vi "spindle_power_save.vi"(0 "Byte Stream File in":refnum<file>, 2 "Array":dbl[](array[numeric]), 5 "base path":path, 7 "Record  SS 661":bool, 9 "Boolean 3":bool, 11 "error in (no error)":errorcluster) -> (4 "Byte Stream File out":refnum<file>, 6 "Boolean 2":bool, 15 "error out":errorcluster)   [LabVIEW 2014]
panel:
  out "Array 2":dbl[](array[numeric])
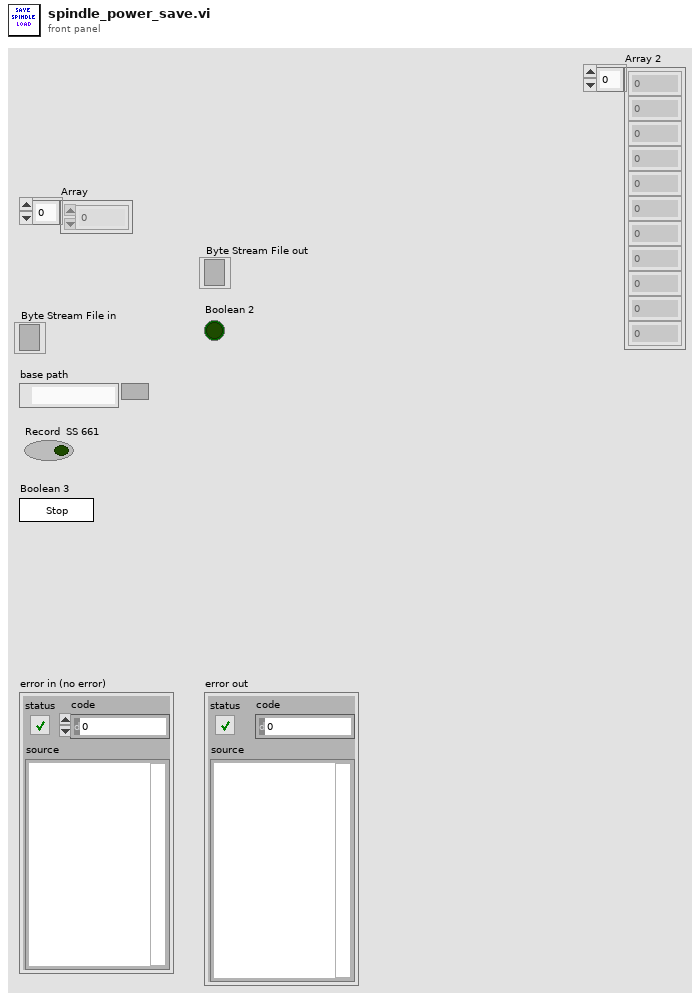
[diagram p1: front panel]
types:
  T1 = enum16{"NotSaving", "Create", "Reading", "Closing"}
  T2 = cluster{"Array":dbl[], "seconds since 1Jan1904":timestamp}
  T3 = enum16{"open", "replace", "create", "open or create", "replace or create", "replace or create with confirmation"}
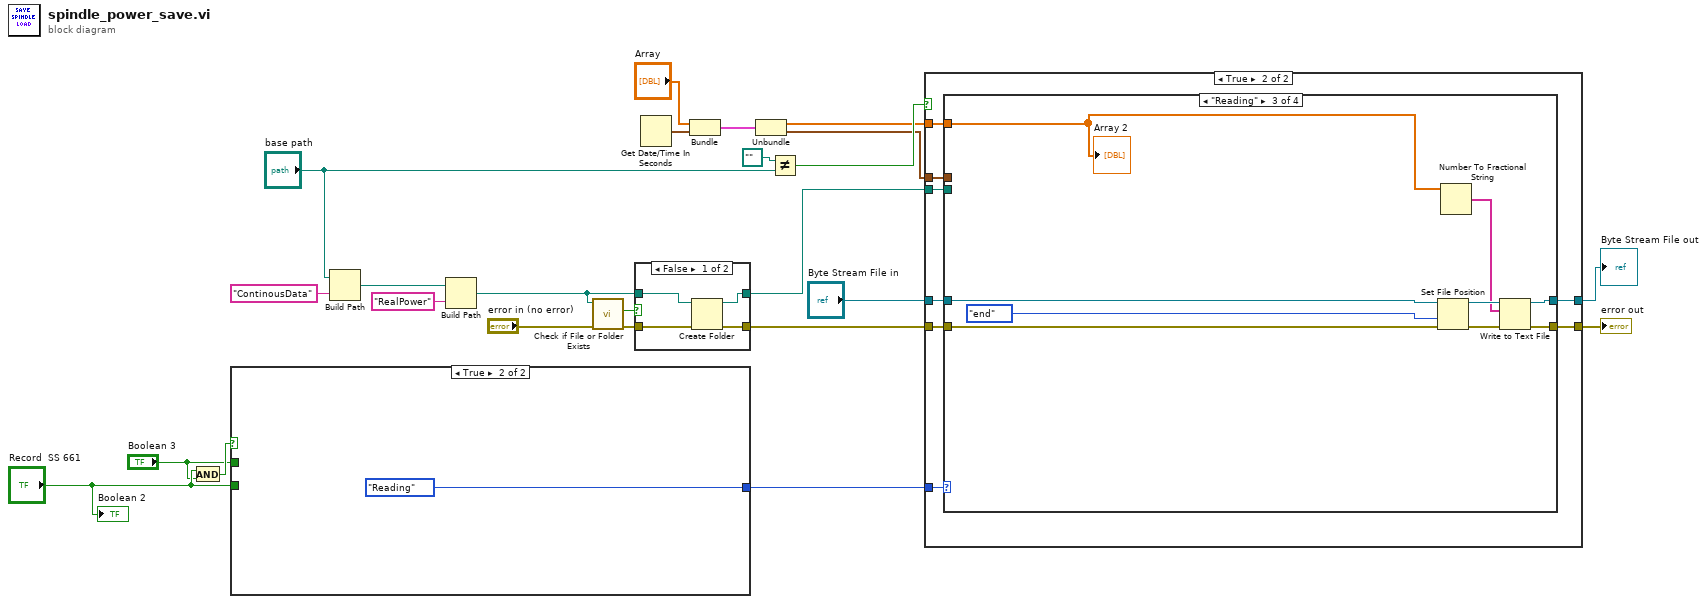
[diagram p0: block diagram]
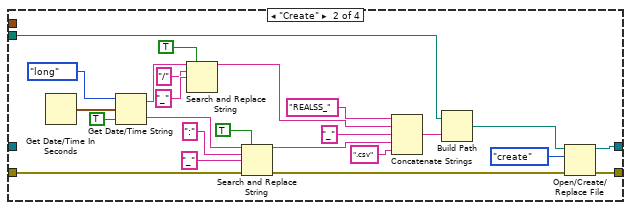
[diagram p5: hidden frame]
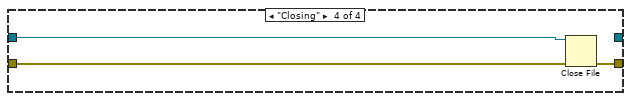
[diagram p6: hidden frame]
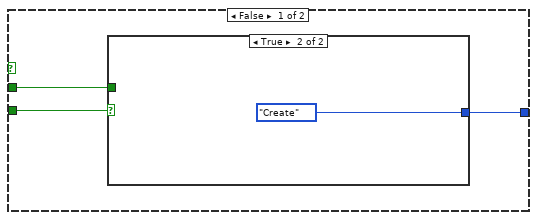
[diagram p7: hidden frame]
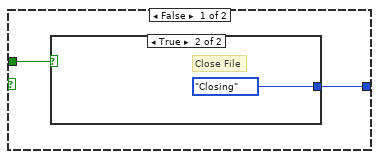
[diagram p8: hidden frame]
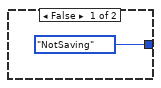
[diagram p9: hidden frame]
diagram:
  n1 = And(x="Record  SS 661", y="Boolean 3") -> (x .and. y?=w18:bool)
  n2 = case shown="True" w18 {
    tunnel: "Boolean 3" -> [w27 _]
    tunnel: [w26 T1."Reading" ("Enum")] -> w17
    tunnel: "Record  SS 661" -> [w25 _]
    frame False {
      n3 = case shown="True" w25 {
        tunnel: w27 -> [w29 _]
        tunnel: [w28 T1."Create" ("Enum")] -> w26
        frame False {
          n4 = case shown="True" w29 {
            tunnel: [T1."NotSaving" ("Enum") T1."Closing" ("Enum")] -> w28
            frame False {
            }
            frame True {
              # "Close File"
            }
          }
        }
        frame True {
        }
      }
    }
    frame True {
    }
  }
  n5 = Build Path(base path="base path", name or relative path="ContinousData") -> (appended path=w9:path)
  n6 = Build Path(base path=w9, name or relative path="RealPower") -> (appended path=w8:path)
  n7 = call <vilib>:"Check if File or Folder Exists.vi"("error in (no error)"="error in (no error)", "path"=w8) -> ("error out"=w11:errorcluster, "file or folder exists?"=w12:bool)  [unwired: 7 in, 1 out]
  n8 = case shown="False" w12 {
    tunnel: [w37 w39] -> w6
    tunnel: w11 -> [w36 w39]
    tunnel: w8 -> [w35 w38]
    tunnel: [w34 w38] -> w7
    frame False {
      n9 = Create Folder(path (use dialog)=w35, error in=w36) -> (created path=w34:path, error out=w37:errorcluster)  [unwired: 1 in, 1 out]
    }
    frame True {
    }
  }
  n10 = Get Date/Time In Seconds() -> (seconds since 1Jan1904=w5:timestamp)
  n11 = Bundle("Array"="Array", "seconds since 1Jan1904"=w5) -> (w4:T2)  [unwired: 1 in]
  n12 = Unbundle(w4) -> ("Array"=w2:dbl[], "seconds since 1Jan1904"=w3:timestamp)
  n13 = Not Equal?(x=path "" ("Project Folder"), y="base path") -> (x != y?=w13:bool)
  n14 = case shown="True" w13 {
    tunnel: w7 -> [_ w46]
    tunnel: w2 -> [_ w48]
    tunnel: w17 -> [_ w47]
    tunnel: w6 -> [w40 w45]
    tunnel: "Byte Stream File in" -> [_ w44]
    tunnel: [_ w43] -> w23
    tunnel: [w40 w42] -> w16
    tunnel: w3 -> [_ w41]
    frame False {
    }
    frame True {
      n15 = case shown="\"Reading\"" w47 {
        tunnel: w48 -> [_ _ w76 _]
        tunnel: w46 -> [_ w74 _ _]
        tunnel: w45 -> [w50 w55 w79 w86]
        tunnel: w44 -> [w49 _ w82 w84]
        tunnel: [w49 w53 w77 _] -> w43
        tunnel: [w50 w52 w78 w85] -> w42
        tunnel: w41 -> [_ _ _ _]
        frame "NotSaving", Default {
        }
        frame "Create" {
          n16 = Get Date/Time In Seconds() -> (seconds since 1Jan1904=w71:timestamp)
          n17 = Get Date/Time String(date format (0)=enum16{"short", "long", "abbreviated"}."long", seconds (now)=w71, want seconds? (F)=TRUE) -> (date string=w69:string, time string=w65:string)
          n18 = Search and Replace String(replace all?=TRUE ("replace all? (F)"), input string=w69, search string="/", replace string="_" ("replace string (\"\")")) -> (result string=w62:string)  [unwired: 4 in, 3 out]
          n19 = Search and Replace String(replace all?=TRUE ("replace all? (F)"), input string=w65, search string=":", replace string="_" ("replace string (\"\")"), error in=w55) -> (result string=w60:string, error out=w56:errorcluster)  [unwired: 3 in, 2 out]
          n20 = Concatenate Strings("REALSS_" ("string"), w62, "_" ("string"), w60, ".csv" ("string")) -> (w58:string)
          n21 = Build Path(base path=w74, name or relative path=w58) -> (appended path=w73:path)
          n22 = Open/Create/Replace File(file path (use dialog)=w73, error in=w56, operation (0:open)=T3."create") -> (refnum out=w53:refnum<file>, error out=w52:errorcluster)  [unwired: 3 in, 1 out]
        }
        frame "Reading" {
          n23 = Set File Position(refnum=w82, from (0:start)=enum16{"start", "end", "current"}."end", error in=w79) -> (refnum out=w81:refnum<file>, error out=w80:errorcluster)  [unwired: 1 in]
          n24 = Number To Fractional String(number=w76) -> (F-format string=w75:string[])  [unwired: 3 in]
          n25 = Write to Text File(file (use dialog)=w81, text=w75, error in=w80) -> (refnum out=w77:refnum<file>, error out=w78:errorcluster)  [unwired: 1 in, 1 out]
          "Array 2" <- w76
        }
        frame "Closing" {
          n26 = Close File(refnum=w84, error in=w86) -> (error out=w85:errorcluster)  [unwired: 1 out]
        }
      }
    }
  }
  "error out" <- w16
  "Byte Stream File out" <- w23
  "Boolean 2" <- "Record  SS 661"
